vi "svfa_Reset Averaging State Info.vi"(0 "f0":dbl, 1 "processing control":T3(ring), 5 "df":dbl, 7 "averaging parameters":T1, 12 "averaging state info in":T2={"complex FFT"=[], "real FFT"=[], "f0"=0.0, "df"=0.0, "averages completed"=0.0, "averaging parameters"={"averaging mode"=enum."No averaging", "weighting mode"=enum."Linear", "number of averages"=10, "linear mode"=enum."Auto restart"}} {"averages completed" format="%.2f"; "df" format="%.2f"; "f0" format="%.2f"; "real FFT" format="%.2f"; "complex FFT" format="%.2f"}) -> (8 "dup averaging parameters":T1, 14 "averaging state info out":T2={"complex FFT"=[], "real FFT"=[], "f0"=0.0, "df"=0.0, "averages completed"=0.0, "averaging parameters"={"averaging mode"=enum."No averaging", "weighting mode"=enum."Linear", "number of averages"=10, "linear mode"=enum."Auto restart"}} {"averages completed" format="%.2f"; "df" format="%.2f"; "f0" format="%.2f"; "real FFT" format="%.2f"; "complex FFT" format="%.2f"})   [LabVIEW 2017]
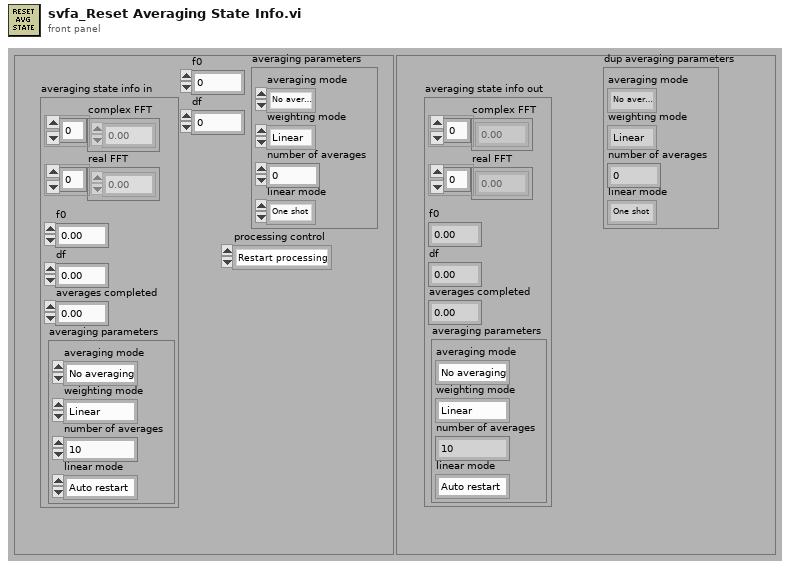
[diagram p1: front panel]
types:
  T1 = cluster{"averaging mode":enum16{"No averaging", "Vector averaging", "RMS averaging", "Peak hold"}, "weighting mode":enum16{"Linear", "Exponential"}, "number of averages":u32, "linear mode":enum16{"One shot", "Auto restart"}}
  T2 = cluster{"complex FFT":cdb[], "real FFT":dbl[], "f0":dbl, "df":dbl, "averages completed":dbl, "averaging parameters":cluster{"averaging mode":enum16{"No averaging", "Vector averaging", "RMS averaging", "Peak hold"}, "weighting mode":enum16{"Linear", "Exponential"}, "number of averages":u32, "linear mode":enum16{"One shot", "Auto restart"}}}
  T3 = enum16{"Restart processing", "Continue processing", "Skip processing"}
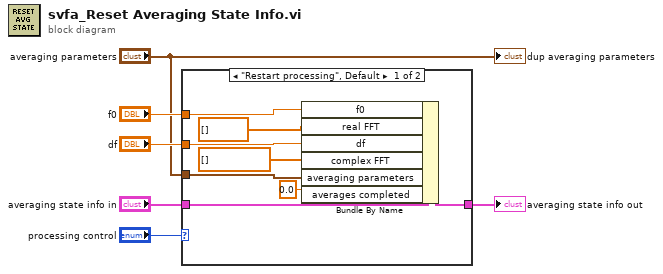
[diagram p0: block diagram]
diagram:
  n1 = case shown="\"Restart processing\", Default" "processing control" {
    tunnel: "averaging state info in" -> [w14 w15]
    tunnel: [w13 w15] -> w5
    tunnel: "f0" -> [w11 _]
    tunnel: "df" -> [w10 _]
    tunnel: "averaging parameters" -> [w7 _]
    frame "Restart processing", Default {
      n2 = Bundle By Name(cluster=w14, "f0"=w11, "real FFT"=dbl[] [], "df"=w10, "complex FFT"=cdb[] [], "averaging parameters"=w7, "averages completed"=0.0) -> (w13:T2)
    }
    frame "Continue processing", "Skip processing" {
    }
  }
  "averaging state info out" <- w5
  "dup averaging parameters" <- "averaging parameters"
